vi "libssh2_session_get_blocking - blocking - returns true.vi"() -> ()   [LabVIEW 2013, in "libssh2_tests.lvlib"]
uses:
  libssh2_tests.lvlib
  libssh2/libssh2_init_default.vi
  <vilib>/addons/_JKI Toolkits/Caraya/classes/Assert/Assert True.vi
  <vilib>/addons/_JKI Toolkits/Caraya/classes/Test/Test.lvclass
  libssh2/libssh2.lvlib
  <vilib>/addons/_JKI Toolkits/Caraya/classes/Assert/Assert.lvclass
panel:
  out "error out":errorcluster
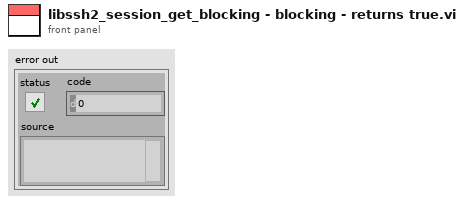
[diagram p1: front panel]
types:
  T1 = typedef "libssh2.lvlib/Session Refnum.ctl" = refnum<k1>
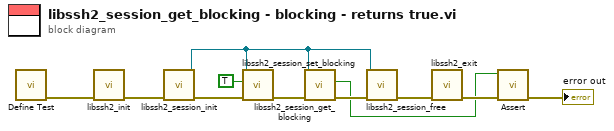
[diagram p0: block diagram]
diagram:
  n1 = call <vilib>:"Define Test.vi"() -> ("error out"=w5:errorcluster)  [unwired: 10 in, 1 out]
  n2 = call-poly "libssh2_init.vi"("error in (no error)"=w5) -> ("error out"=w9:errorcluster)  [unwired: 10 in]
  n3 = call "libssh2_session_init.vi"("error in (no error)"=w9) -> ("error out"=w10:errorcluster, "session"=w2:T1)  [unwired: 9 in]
  n4 = call "libssh2_session_set_blocking.vi"("error in (no error)"=w10, "blocking"=TRUE, "session"=w2) -> ("error out"=w7:errorcluster)  [unwired: 8 in]
  n5 = call "libssh2_session_get_blocking.vi"("error in (no error)"=w7, "session"=w2) -> ("error out"=w3:errorcluster, "blocking"=w1:bool)  [unwired: 8 in]
  n6 = call "libssh2_session_free.vi"("error in (no error)"=w3, "session"=w2) -> ("error out"=w8:errorcluster)  [unwired: 9 in]
  n7 = call "libssh2_exit.vi"("error in (no error)"=w8) -> ("error out"=w6:errorcluster)  [unwired: 10 in]
  n8 = call-poly <vilib>:"Assert.vi"("error in (no error)"=w6, "True?"=w1) -> ("error out"=→"error out":errorcluster)  [unwired: 8 in, 1 out]
